vi "CRYGet Window Array.vi"(9 "size(s)":i32, 10 "Fs":dbl, 11 "TSR Window Name":string) -> (3 "Window Array":dbl[](array[numeric]))   [LabVIEW 2013]
uses:
  <vilib>/Analysis/4window.llb/windowTd.ctl
  <vilib>/Analysis/4window.llb/Cosine Tapered Window (DBL).vi
  <vilib>/Analysis/4window.llb/Exponential Window (DBL).vi
  <vilib>/Analysis/4window.llb/Blackman-Harris Window (DBL).vi
  <vilib>/Analysis/4window.llb/AllCosWindow (DBL).vi
  <vilib>/Analysis/0measdsp.llb/Scaled Time Domain Window (DBL).vi
  <vilib>/Analysis/NI_AALPro.lvlib
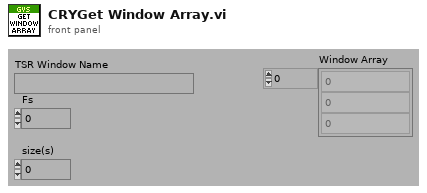
[diagram p1: front panel]
types:
  T1 = typedef "NI_AALPro.lvlib/windowTd.ctl" = u32
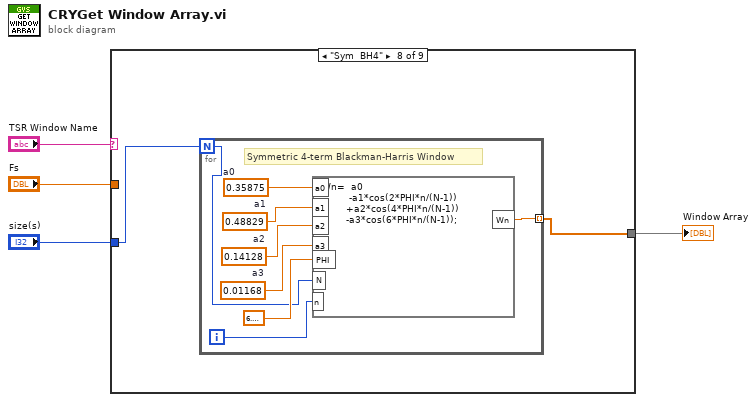
[diagram p0: block diagram]
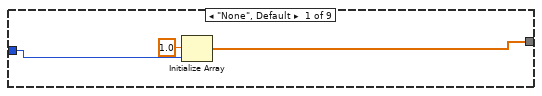
[diagram p2: hidden frame]
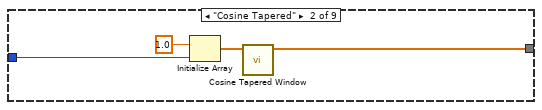
[diagram p3: hidden frame]
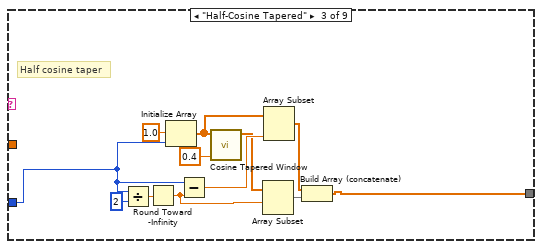
[diagram p4: hidden frame]
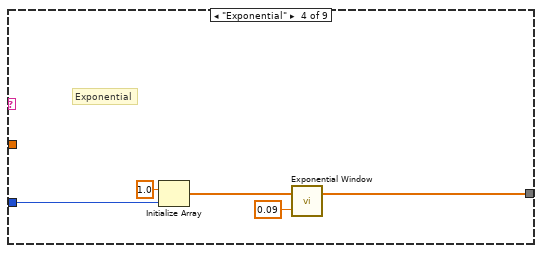
[diagram p5: hidden frame]
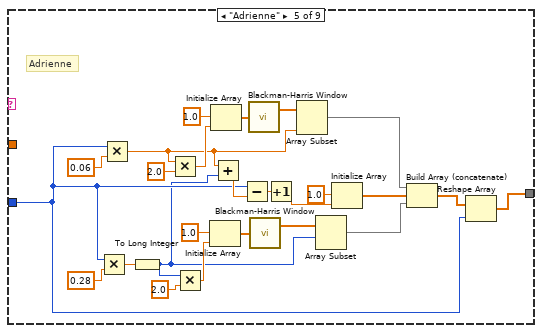
[diagram p6: hidden frame]
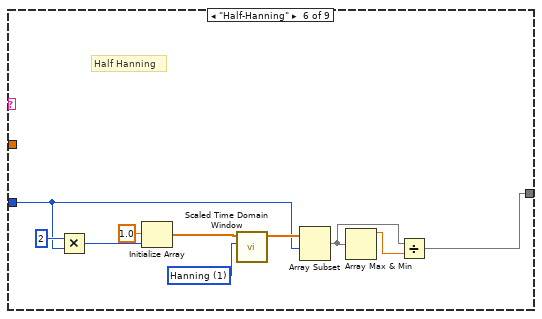
[diagram p7: hidden frame]
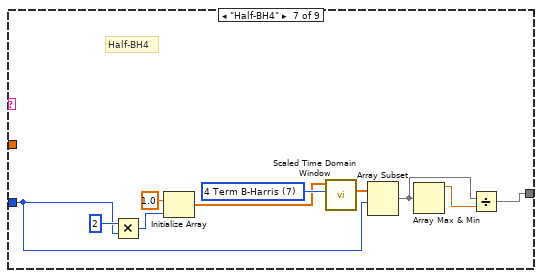
[diagram p8: hidden frame]
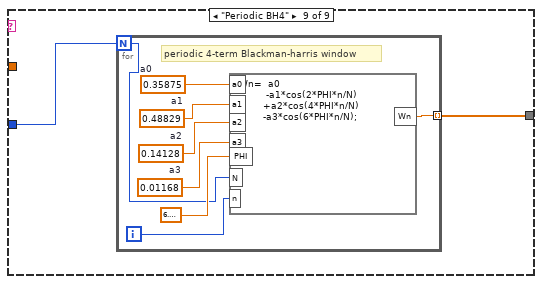
[diagram p9: hidden frame]
diagram:
  n1 = case shown="\"Sym  BH4\"" "TSR Window Name" {
    tunnel: "Fs" -> [_ _ _ _ _ _ _ _ _]
    tunnel: [w5 w8 w12 w25 w35 w54 w64 w74 w84] -> w1
    tunnel: "size(s)" -> [w6 w10 w13 w24 w34 w56 w67 w75 w85]
    frame "None", Default {
      n2 = Initialize Array(1.0 ("element"), w6) -> (w5:dbl[])
    }
    frame "Cosine Tapered" {
      n3 = Initialize Array(1.0 ("element"), w10) -> (w9:dbl[])
      n4 = call-poly <vilib>:"Cosine Tapered Window.vi"("X"=w9) -> ("Windowed X"=w8:dbl[])  [unwired: 1 in, 9 out]
    }
    frame "Half-Cosine Tapered" {
      # "Half cosine taper"
      n5 = Divide(x=w13, y=2) -> (x/y=w22:dbl)
      n6 = Round Toward -Infinity(1:w22) -> (0:w20:dbl)
      n7 = Initialize Array(1.0 ("element"), w13) -> (w18:dbl[])
      n8 = Subtract(x=w13, y=w20) -> (x-y=w16:dbl)
      n9 = call-poly <vilib>:"Cosine Tapered Window.vi"("ratio"=0.4, "X"=w18) -> ("Windowed X"=w14:dbl[])  [unwired: 8 in, 1 out]
      n10 = Array Subset(array=w14, index=w20) -> (w19:dbl[])  [unwired: 1 in]
      n11 = Array Subset(array=w18, length=w16) -> (w17:dbl[])  [unwired: 1 in]
      n12 = Build Array (concatenate)(w17, w19) -> (w12:dbl[])
    }
    frame "Exponential" {
      # "Exponential"
      n13 = Initialize Array(1.0 ("element"), w24) -> (w27:dbl[])
      n14 = call-poly <vilib>:"Exponential Window.vi"("final value"=0.09, "X"=w27) -> ("Windowed X"=w25:dbl[])  [unwired: 1 out]
    }
    frame "Adrienne" {
      # "Adrienne"
      n15 = Multiply(x=w34, y=0.28) -> (x*y=w33:dbl)
      n16 = Multiply(x=w34, y=0.06) -> (x*y=w38:dbl)
      n17 = To Long Integer(number=w33) -> (32bit integer=w31:i32)
      n18 = Multiply(x=w38, y=2.0) -> (x*y=w45:dbl)
      n19 = Multiply(x=w31, y=2.0) -> (x*y=w32:dbl)
      n20 = Initialize Array(1.0 ("element"), w32) -> (w41:dbl[])
      n21 = Initialize Array(1.0 ("element"), w45) -> (w52:dbl[])
      n22 = Add(x=w38, y=w31) -> (x+y=w37:dbl)
      n23 = Subtract(x=w34, y=w37) -> (x-y=w46:dbl)
      n24 = call-poly <vilib>:"Blackman-Harris Window.vi"("X"=w52) -> ("Windowed X"=w29:dbl[])  [unwired: 1 out]
      n25 = call-poly <vilib>:"Blackman-Harris Window.vi"("X"=w41) -> ("Windowed X"=w40:dbl[])  [unwired: 1 out]
      n26 = Increment(x=w46) -> (x+1=w30:dbl)
      n27 = Array Subset(array=w29, length=w38) -> (w48:dbl[])  [unwired: 1 in]
      n28 = Array Subset(array=w40, index=w31) -> (w39:dbl[])  [unwired: 1 in]
      n29 = Initialize Array(1.0 ("element"), w30) -> (w49:dbl[])
      n30 = Build Array (concatenate)(w48, w49, w39) -> (w36:dbl[])
      n31 = Reshape Array(w36, w34) -> (w35:dbl[])
    }
    frame "Half-Hanning" {
      w60 = T1 1 items=["Rectangle"=0, "Hanning"=1, "Hamming"=2, "Blackman-Harris"=3, "Exact Blackman"=4, "Blackman"=5, "Flat Top"=6, "4 Term B-Harris "=7, "7 Term B-Harris"=8, "Low Sidelobe"=9, "Blackman Nuttall"=11, "Triangle"=30, "Bartlett-Hanning"=31, "Bohman"=32, "Parzen"=33, "Welch"=34, "Kaiser"=60, "Dolph-Chebyshev"=61, "Gaussian"=62] ("window")
      # "Half Hanning"
      n32 = Multiply(x=2, y=w56) -> (x*y=w61:i32)
      n33 = Initialize Array(1.0 ("element"), w61) -> (w58:dbl[])
      n34 = call-poly <vilib>:"Scaled Time Domain Window.vi"("window"=w60, "X"=w58) -> ("Windowed X"=w57:dbl[])  [unwired: 7 in, 2 out]
      n35 = Array Subset(array=w57, index=w56) -> (w55:dbl[])  [unwired: 1 in]
      n36 = Array Max & Min(array=w55) -> (max value=w59:dbl)  [unwired: 3 out]
      n37 = Divide(x=w55, y=w59) -> (x/y=w54:dbl[])
    }
    frame "Half-BH4" {
      w71 = T1 7 items=["Rectangle"=0, "Hanning"=1, "Hamming"=2, "Blackman-Harris"=3, "Exact Blackman"=4, "Blackman"=5, "Flat Top"=6, "4 Term B-Harris "=7, "7 Term B-Harris"=8, "Low Sidelobe"=9, "Blackman Nuttall"=11, "Triangle"=30, "Bartlett-Hanning"=31, "Bohman"=32, "Parzen"=33, "Welch"=34, "Kaiser"=60, "Dolph-Chebyshev"=61, "Gaussian"=62] ("window")
      # "Half-BH4"
      n38 = Multiply(x=2, y=w67) -> (x*y=w69:i32)
      n39 = Initialize Array(1.0 ("element"), w69) -> (w70:dbl[])
      n40 = call-poly <vilib>:"Scaled Time Domain Window.vi"("window"=w71, "X"=w70) -> ("Windowed X"=w68:dbl[])  [unwired: 7 in, 2 out]
      n41 = Array Subset(array=w68, index=w67) -> (w65:dbl[])  [unwired: 1 in]
      n42 = Array Max & Min(array=w65) -> (max value=w66:dbl)  [unwired: 3 out]
      n43 = Divide(x=w65, y=w66) -> (x/y=w64:dbl[])
    }
    frame "Sym  BH4" {
      n44 = for {
        N: w75 -> [w77]
        tunnel: [w78] -> w74 mode=indexing
        i -> [w76]
        w80 = 0.01168  # a3
        w81 = 0.14128  # a2
        w82 = 0.48829  # a1
        w83 = 0.35875  # a0
        # "Symmetric 4-term Blackman-Harris Window"
        n45 = formula code="Wn=  a0\n         -a1*cos(2*PHI*n/(N-1))\n        +a2*cos(4*PHI*n/(N-1))\n        -a3*cos(6*PHI*n/(N-1));"("a0"=w83, "a1"=w82, "a2"=w81, "a3"=w80, "PHI"=6.283185307179586, "N"=w77, "n"=w76) -> ("Wn"=w78:dbl)
      }
    }
    frame "Periodic BH4" {
      n46 = for {
        N: w85 -> [w87]
        tunnel: [w88] -> w84 mode=indexing
        i -> [w86]
        w90 = 0.01168  # a3
        w91 = 0.14128  # a2
        w92 = 0.48829  # a1
        w93 = 0.35875  # a0
        # "periodic 4-term Blackman-harris window"
        n47 = formula code="Wn=  a0\n         -a1*cos(2*PHI*n/N)\n        +a2*cos(4*PHI*n/N)\n        -a3*cos(6*PHI*n/N);"("a0"=w93, "a1"=w92, "a2"=w91, "a3"=w90, "PHI"=6.283185307179586, "N"=w87, "n"=w86) -> ("Wn"=w88:dbl)
      }
    }
  }
  "Window Array" <- w1
